vi "Test1_2.vi"(0 "Instrument VISA in":T1={"AWG VISA"="81160A", "Oscilloscope  VISA "="DSO80204B", "Integration Board IP"="172.16.7.43", "connection ID"=refnum, "report out"=refnum}, 2 "Report Enable":bool, 5 "DT_50_L0":i32[][](array[numeric]), 7 "Cycles Burst":i32=10000, 9 "Voltage Step":dbl, 11 "error in":errorcluster) -> (4 "Instrument VISA out":T1={"AWG VISA"="81160A", "Oscilloscope  VISA "="DSO80204B", "Integration Board IP"="172.16.7.43", "connection ID"=refnum, "report out"=refnum}, 6 "StDev":dbl[][](array[numeric]), 10 "XY Graph":cluster{"Y":dbl[], "Y":dbl[]}[](graph), 15 "error out":errorcluster)   [LabVIEW 2009]
doc: "This VI provides the distribution of the detected IPR using different pulse amplitudes."
uses:
  <vilib>/Utility/NIReport.llb/NI_report.lvclass
  <vilib>/Utility/NIReport.llb/Append Text Table to Report (wrap).vi
  <vilib>/Utility/NIReport.llb/Append Report Text (str wrap).vi
  <instrlib>/Agilent 81150/Agilent 81150.lvlib
  <vilib>/gmath/NI_Gmath.lvlib
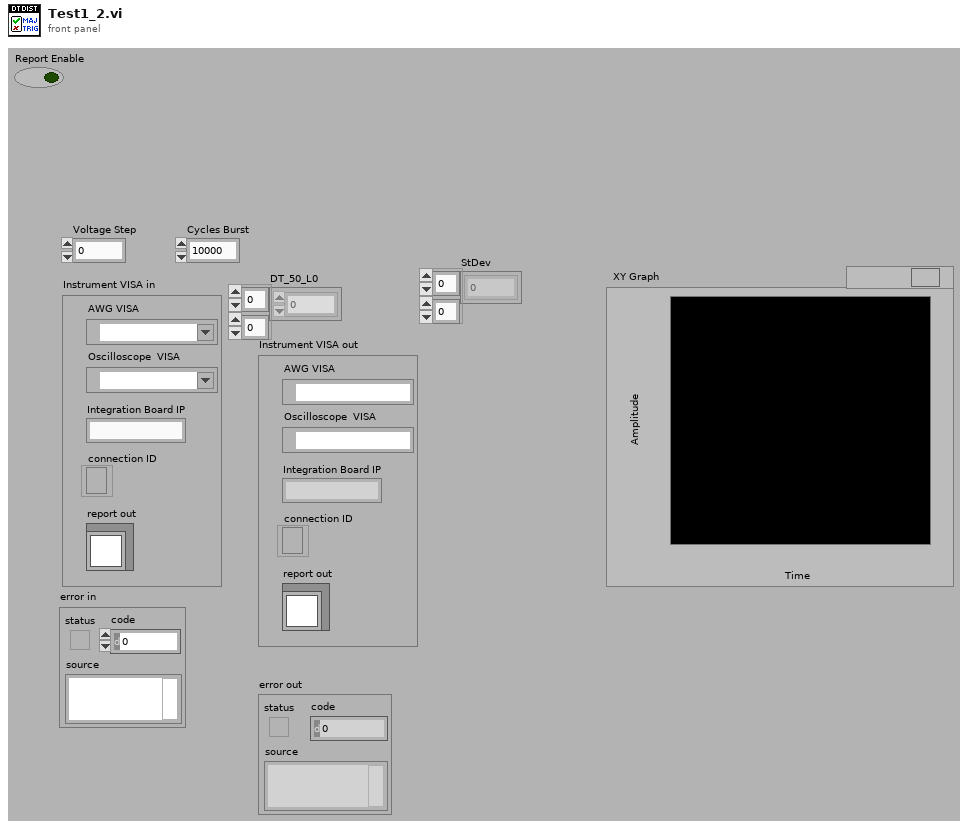
[diagram p1: front panel]
types:
  T1 = cluster{"AWG VISA":refnum<visa-resource-name>, "Oscilloscope  VISA ":refnum<visa-resource-name>, "Integration Board IP":string, "connection ID":refnum<k5>, "report out":refnum<class "NI_report.lvclass">}
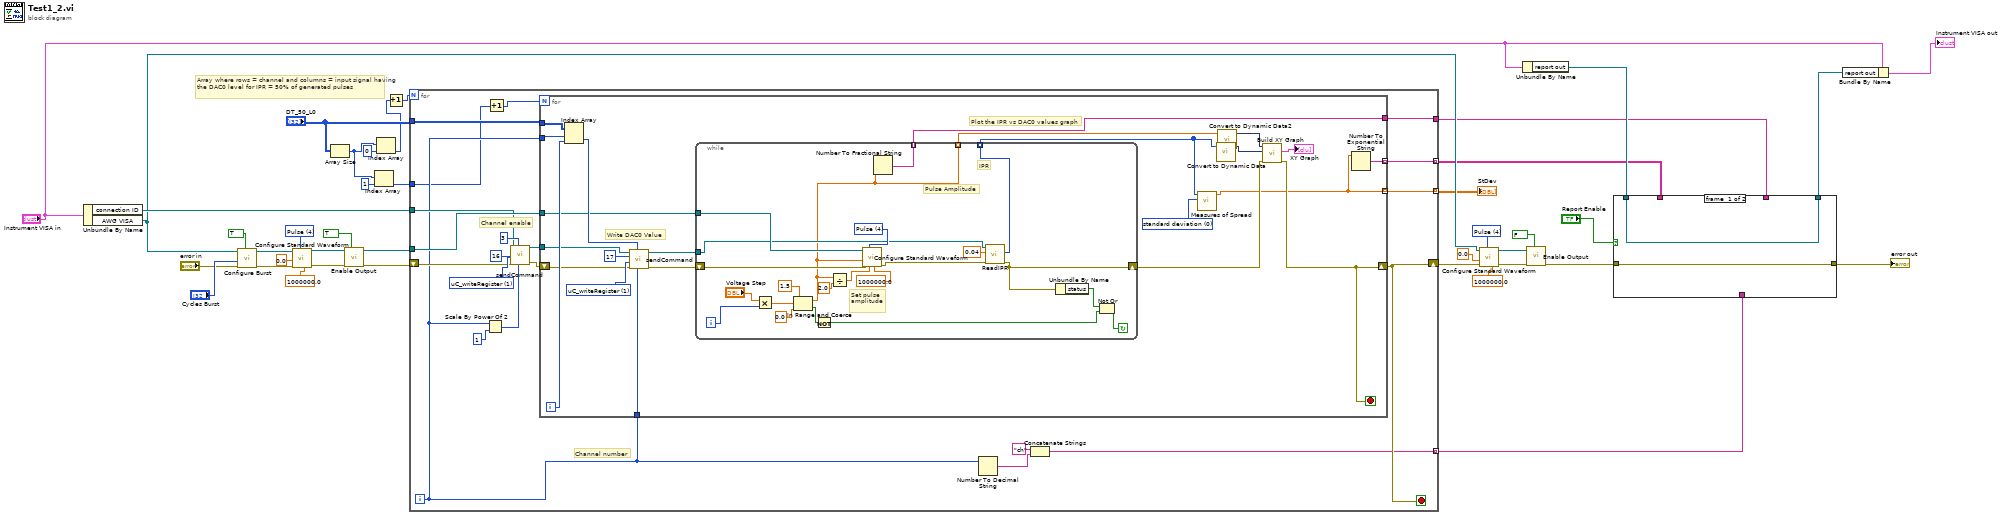
[diagram p0: block diagram]
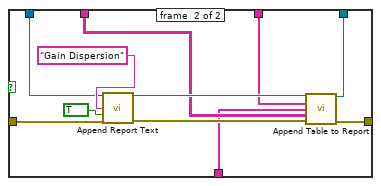
[diagram p2: hidden frame]
diagram:
  w26 = u16 4 items=["Sine", "Square", "Ramp Up", "Ramp Down", "Pulse", "Noise", "DC"] ("Waveform (0: Sine)")
  w39 = u16 4 items=["Sine", "Square", "Ramp Up", "Ramp Down", "Pulse", "Noise", "DC"] ("Waveform (0: Sine)")
  # "Array where rows = channel and columns = input signal having the DAC0 level for IPR = 50% of generated pulses"
  n1 = Unbundle By Name("Instrument VISA in") -> ("connection ID"=w29:refnum<k5>, "AWG VISA"=w20:refnum<visa-resource-name>)
  n2 = call <instrlib>:"Configure Burst.vi"("Enable Burst (F: Disable)"=TRUE, "error in (no error)"="error in", "Burst Count (2)"="Cycles Burst", "VISA resource name"=w20) -> ("error out"=w36:errorcluster, "VISA resource name out"=w37:refnum<visa-resource-name>)  [unwired: 6 in]
  n3 = call <instrlib>:"Configure Standard Waveform.vi"("Frequency (1000.0 Hz)"=1000000.0, "Waveform (0: Sine)"=w39, "error in (no error)"=w36, "Amplitude (1.0 Vpp)"=0.0, "VISA resource name"=w37) -> ("error out"=w35:errorcluster, "VISA resource name out"=w34:refnum<visa-resource-name>)  [unwired: 5 in]
  n4 = Array Size(array="DT_50_L0") -> (size(s)=w5:i32[])
  n5 = call <instrlib>:"Enable Output.vi"("Enable Output (T: Enable)"=TRUE, "error in (no error)"=w35, "VISA resource name"=w34) -> ("error out"=w30:errorcluster, "VISA resource name out"=w28:refnum<visa-resource-name>)  [unwired: 7 in]
  n6 = Index Array(array=w5, index=1) -> (element=w3:i32)
  n7 = Index Array(array=w5, index=0) -> (element=w1:i32)
  n8 = Increment(x=w1) -> (x+1=w2:i32)
  n9 = for {
    N: w2 -> [_]
    shift-right: [w54] -> w22
    shift-left: w30 -> [w58]
    tunnel: w28 -> [w52]
    tunnel: w29 -> [w51]
    tunnel: "DT_50_L0" -> [w50]
    tunnel: [w49] -> w19 mode=indexing
    tunnel: [w48] -> w13 mode=indexing
    tunnel: [w44] -> w12 mode=indexing
    tunnel: [w43] -> w11
    tunnel: w3 -> [w41]
    i -> [w45]
    stop <- w54 stop-if-true
    w61 = u16 1 items=["sendCommand"=9, "FPGA_writeRegister"=3, "FPGA_readRegister"=2, "uC_writeRegister"=1, "uC_readRegister"=0] ("Action")
    # "Channel number"
    # "Channel enable"
    n10 = Scale By Power Of 2(n=w45, x=1) -> (x*2^n=w56:i32)
    n11 = Increment(x=w41) -> (x+1=w42:i32)
    n12 = call "sendCommand.vi"("Address"=w56, "Data"=3, "error in"=w58, "Action"=w61, "id"=16, "connection ID"=w51) -> ("error out"=w55:errorcluster, "connection ID out"=w53:refnum<k5>)  [unwired: 2 in, 2 out]
    n13 = for {
      N: w42 -> [_]
      shift-right: [w68] -> w54
      shift-left: w55 -> [w75]
      tunnel: w53 -> [w67]
      tunnel: w52 -> [w65]
      tunnel: w50 -> [w77]
      tunnel: w45 -> [w78]
      tunnel: w45 -> [w74]
      tunnel: [w64] -> w49 mode=indexing
      tunnel: [w63] -> w48 mode=indexing
      tunnel: [w62] -> w43
      i -> [w76]
      stop <- w68 stop-if-true
      w71 = 0 items=["standard deviation", "range", "mean absolute deviation", "interquartile range"] ("type")
      w80 = u16 1 items=["sendCommand"=9, "FPGA_writeRegister"=3, "FPGA_readRegister"=2, "uC_writeRegister"=1, "uC_readRegister"=0] ("Action")
      # "Write DAC0 Value"
      # "Plot the IPR vs DAC0 values graph"
      n14 = Index Array(array=w77, index (row)=w78, index (col)=w76) -> (element=w73:i32)
      n15 = call "sendCommand.vi"("Address"=w74, "Data"=w73, "error in"=w75, "Action"=w80, "id"=17, "connection ID"=w67) -> ("error out"=w72:errorcluster, "connection ID out"=w66:refnum<k5>)  [unwired: 2 in, 2 out]
      n16 = while {
        tunnel: [w89] -> w70 mode=indexing
        tunnel: [w87] -> w82 mode=indexing
        shift-right: [w92] -> w69
        shift-left: w72 -> [w99]
        tunnel: w66 -> [w91]
        tunnel: w65 -> [w94]
        tunnel: [w88] -> w62 mode=indexing
        i -> [w98]
        stop <- w95 continue-if-true
        w101 = u16 4 items=["Sine", "Square", "Ramp Up", "Ramp Down", "Pulse", "Noise", "DC"] ("Waveform (0: Sine)")
        # "Set pulse amplitude"
        # "IPR"
        # "Pulse Amplitude"
        n17 = Multiply(x="Voltage Step", y=w98) -> (x*y=w105:dbl)
        n18 = In Range and Coerce(upper limit=1.5, x=w105, lower limit=0.0) -> (coerced(x)=w87:dbl, In Range?=w106:bool)
        n19 = Not(x=w106) -> (.not. x?=w96:bool)
        n20 = Divide(x=w87, y=2.0) -> (x/y=w85:dbl)
        n21 = call <instrlib>:"Configure Standard Waveform.vi"("Frequency (1000.0 Hz)"=1000000.0, "DC Offset (0.0 Volts)"=w85, "Waveform (0: Sine)"=w101, "error in (no error)"=w99, "Amplitude (1.0 Vpp)"=w87, "VISA resource name"=w94) -> ("error out"=w93:errorcluster)  [unwired: 4 in, 1 out]
        n22 = Number To Fractional String(number=w87) -> (F-format string=w88:string)  [unwired: 3 in]
        n23 = call "ReadIPR.vi"("error in"=w93, "Delay Time (s)"=0.04, "connection ID"=w91) -> ("error out"=w92:errorcluster, "IPR value"=w89:i32)  [unwired: 6 in, 1 out]
        n24 = Unbundle By Name(w92) -> ("status"=w97:bool)
        n25 = Not Or(1:w96, 2:w97) -> (0:w95:bool)
      }
      n26 = call <vilib>:"Measures of Spread.vi"("type"=w71, "x array"=w70) -> ("spread value"=w64:dbl)  [unwired: 8 in, 1 out]
      n27 = call "Convert to Dynamic Data"("Array"=w70) -> ("Dynamic Data Type"=w83:dynamicdata)  [unwired: 3 in]
      n28 = call "Convert to Dynamic Data2"("Array"=w82) -> ("Dynamic Data Type"=w81:dynamicdata)  [unwired: 3 in]
      n29 = call "Build XY Graph"("error in (no error)"=w69, "Y Input"=w83, "X Input"=w81) -> ("error out"=w68:errorcluster, "XY Graph"=→"XY Graph":cluster{"Y":dbl[], "Y":dbl[]}[])  [unwired: 7 in]
      n30 = Number To Exponential String(number=w64) -> (E-format string=w63:string)  [unwired: 3 in]
    }
    n31 = Number To Decimal String(number=w45) -> (decimal integer string=w46:string)  [unwired: 1 in]
    n32 = Concatenate Strings("ch" ("string"), w46) -> (w44:string)
  }
  "StDev" <- w19
  n33 = call <instrlib>:"Configure Standard Waveform.vi"("Frequency (1000.0 Hz)"=1000000.0, "Waveform (0: Sine)"=w26, "error in (no error)"=w22, "Amplitude (1.0 Vpp)"=0.0, "VISA resource name"=w20) -> ("error out"=w23:errorcluster, "VISA resource name out"=w21:refnum<visa-resource-name>)  [unwired: 5 in]
  n34 = Unbundle By Name("Instrument VISA in") -> ("report out"=w17:refnum<class "NI_report.lvclass">)
  n35 = call <instrlib>:"Enable Output.vi"("Enable Output (T: Enable)"=FALSE, "error in (no error)"=w23, "VISA resource name"=w21) -> ("error out"=w16:errorcluster)  [unwired: 7 in, 1 out]
  n36 = case shown="True" "Report Enable" {
    tunnel: [w107 w119] -> w15
    tunnel: w16 -> [w107 w118]
    tunnel: w17 -> [w108 w113]
    tunnel: w13 -> [_ w112]
    tunnel: [w108 w111] -> w8
    tunnel: w12 -> [_ w110]
    tunnel: w11 -> [_ w109]
    frame #0 {
    }
    frame #1 {
      n37 = call-poly <vilib>:"Append Report Text.vi"("report in"=w113, "text"="Gain Dispersion", "append on new line? (F)"=TRUE, "error in (no error)"=w118) -> ("report out"=w114:refnum<class "NI_report.lvclass">, "error out"=w117:errorcluster)  [unwired: 8 in, 2 out]
      n38 = call-poly <vilib>:"Append Table to Report.vi"("report in"=w114, "column headers"=w109, "row headers"=w110, "text data"=w112, "error in (no error)"=w117) -> ("report out"=w111:refnum<class "NI_report.lvclass">, "error out"=w119:errorcluster)  [unwired: 7 in, 2 out]
    }
  }
  "error out" <- w15
  n39 = Bundle By Name(cluster="Instrument VISA in", "report out"=w8) -> (→"Instrument VISA out":T1)
